vi "Monitor Stop.vi"(8 "error in (no error)":errorcluster, 10 "Actor Data":T1={"Actor Type"="", "Actor Core VI"="", "Self"=refnum, "Caller"=refnum, "Actor Label"="", "Last Ping"=-1.0}, 11 "Orphan Detector in":refnum<class "Orphan Detector.lvclass">) -> (0 "error out":errorcluster, 3 "Orphan Detector out":refnum<class "Orphan Detector.lvclass">)   [LabVIEW 2023, in "Monitored Actor.lvlib" / "Orphan Detector.lvclass"]
doc: "Adds the actor to the list of orphaned actors\n\nCopyright: MGI 2016\nAuthor: Derek Trepanier"
uses:
  Orphan Detector.lvclass
  Monitor Data/Actor Data.ctl
  builds/Engine/Actor Framework.lvlibp/1abvi3w/vi.lib/ActorFramework/Message Enqueuer/Message Enqueuer.lvclass
  builds/Engine/Actor Framework.lvlibp/1abvi3w/vi.lib/ActorFramework/Message/Message.lvclass
  Orphan Detector.lvclass/Orphan Detector.ctl
  Monitor Data/Monitor Data.lvclass
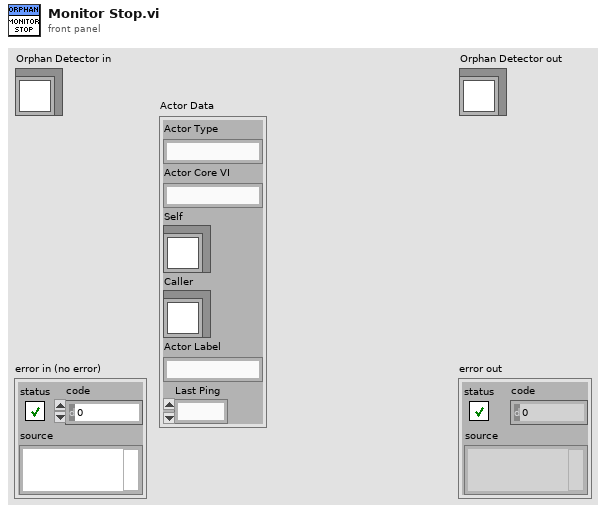
[diagram p1: front panel]
types:
  T1 = typedef "Monitored Actor.lvlib/Monitor Data.lvclass/Actor Data.ctl" = cluster{"Actor Type":string, "Actor Core VI":string, "Self":refnum<class "Message Enqueuer.lvclass">, "Caller":refnum<class "Message Enqueuer.lvclass">, "Actor Label":string, "Last Ping":dbl}
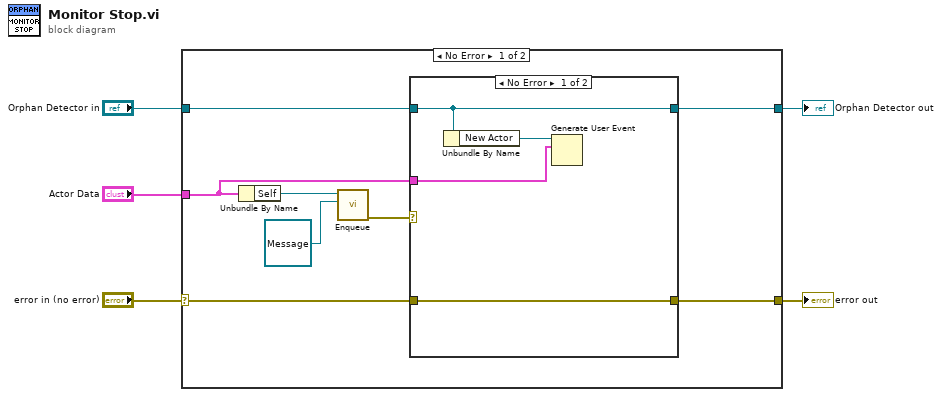
[diagram p0: block diagram]
diagram:
  n1 = case shown="No Error" "error in (no error)" {
    selector: "error in (no error)" -> [w11 w21]
    tunnel: [w7 w21] -> w4
    tunnel: [w9 w20] -> w2
    tunnel: "Orphan Detector in" -> [w8 w20]
    tunnel: "Actor Data" -> [w6 _]
    frame No Error {
      n2 = Unbundle By Name(w6) -> ("Self"=w13:refnum<class "Message Enqueuer.lvclass">)
      n3 = call "Enqueue.vi"("Message"=refnum<class "Message.lvclass"> refnum, "Message Enqueuer in"=w13) -> ("error out"=w10:errorcluster)  [unwired: 8 in, 1 out]
      n4 = case shown="No Error" w10 {
        tunnel: w11 -> [w14 w18]
        tunnel: [w17 w19] -> w9
        tunnel: w8 -> [w17 w19]
        tunnel: [w14 w18] -> w7
        tunnel: w6 -> [w15 _]
        frame No Error {
          n5 = Unbundle By Name(w17) -> ("New Actor"=w16:refnum<user-event>)
          n6 = Generate User Event(user event=w16, event data cluster=w15) -> ()  [unwired: 2 in, 2 out]
        }
        frame Error {
          # "Q already dead, actor is stopped, this actor is in good shape."
        }
      }
    }
    frame Error {
    }
  }
  "error out" <- w4
  "Orphan Detector out" <- w2
